vi "Servo(s) (subVI).vi"(0 "PWM channel 2":tag="B/PWM0", 2 "duty cycle [%]":dbl, 3 "error in (no error)":errorcluster) -> (10 "error out":errorcluster)   [LabVIEW 2017]
uses:
  <vilib>/Utility/error.llb/Error Cluster From Error Code.vi
  <vilib>/myRIO/Instrument Drivers/Onboard IO/PWM/PWM.lvlib
panel:
  in  "Servo stop":bool
  in  "freq [Hz]":dbl=50.0
  # "Servo"
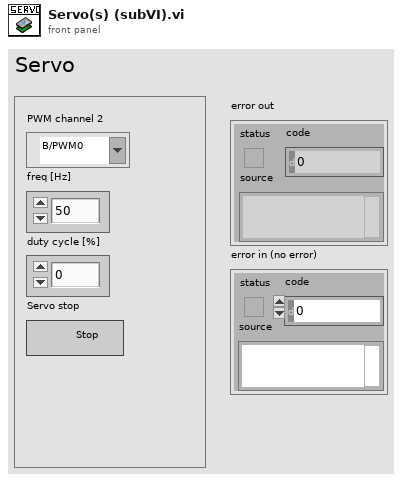
[diagram p1: front panel]
types:
  T1 = typedef "PWM.lvlib/PWM Reference.ctl" = cluster{"myRIO Reference":T2, "PWM Channels Enum":T6, "PWM Configuration":T7}
  T2 = typedef "myRIO Generic Hardware Reference.ctl" = cluster{"myRIO Model":T3, "myRIO Hardware Reference":T4}
  T3 = typedef "Hardware Version Enum.ctl" = enum16{"Unknown", "myRIO-1900", "myRIO-1950", "roboRIO", "NI ELVIS RIO CM"}
  T4 = typedef "myRIO v1.0 Reference.ctl" = cluster{"Generic FPGA Reference":T5, "Allow multiple opens":bool}
  T5 = typedef "Generic FPGA Reference.ctl" = refnum<k20>
  T6 = typedef "PWM Channels Enum.ctl" = enum16{"Not Connected", "C/PWM0", "C/PWM1", "A/PWM0", "A/PWM1", "A/PWM2", "B/PWM0", "B/PWM1", "B/PWM2", "PWM/PWM0", "PWM/PWM1", "PWM/PWM2", "PWM/PWM3", "PWM/PWM4", "PWM/PWM5", "PWM/PWM6", "PWM/PWM7", "PWM/PWM8", "PWM/PWM9"}
  T7 = typedef "PWM.lvlib/PWM Configuration.ctl" = cluster{"Frequency":dbl, "Duty Cycle":dbl}
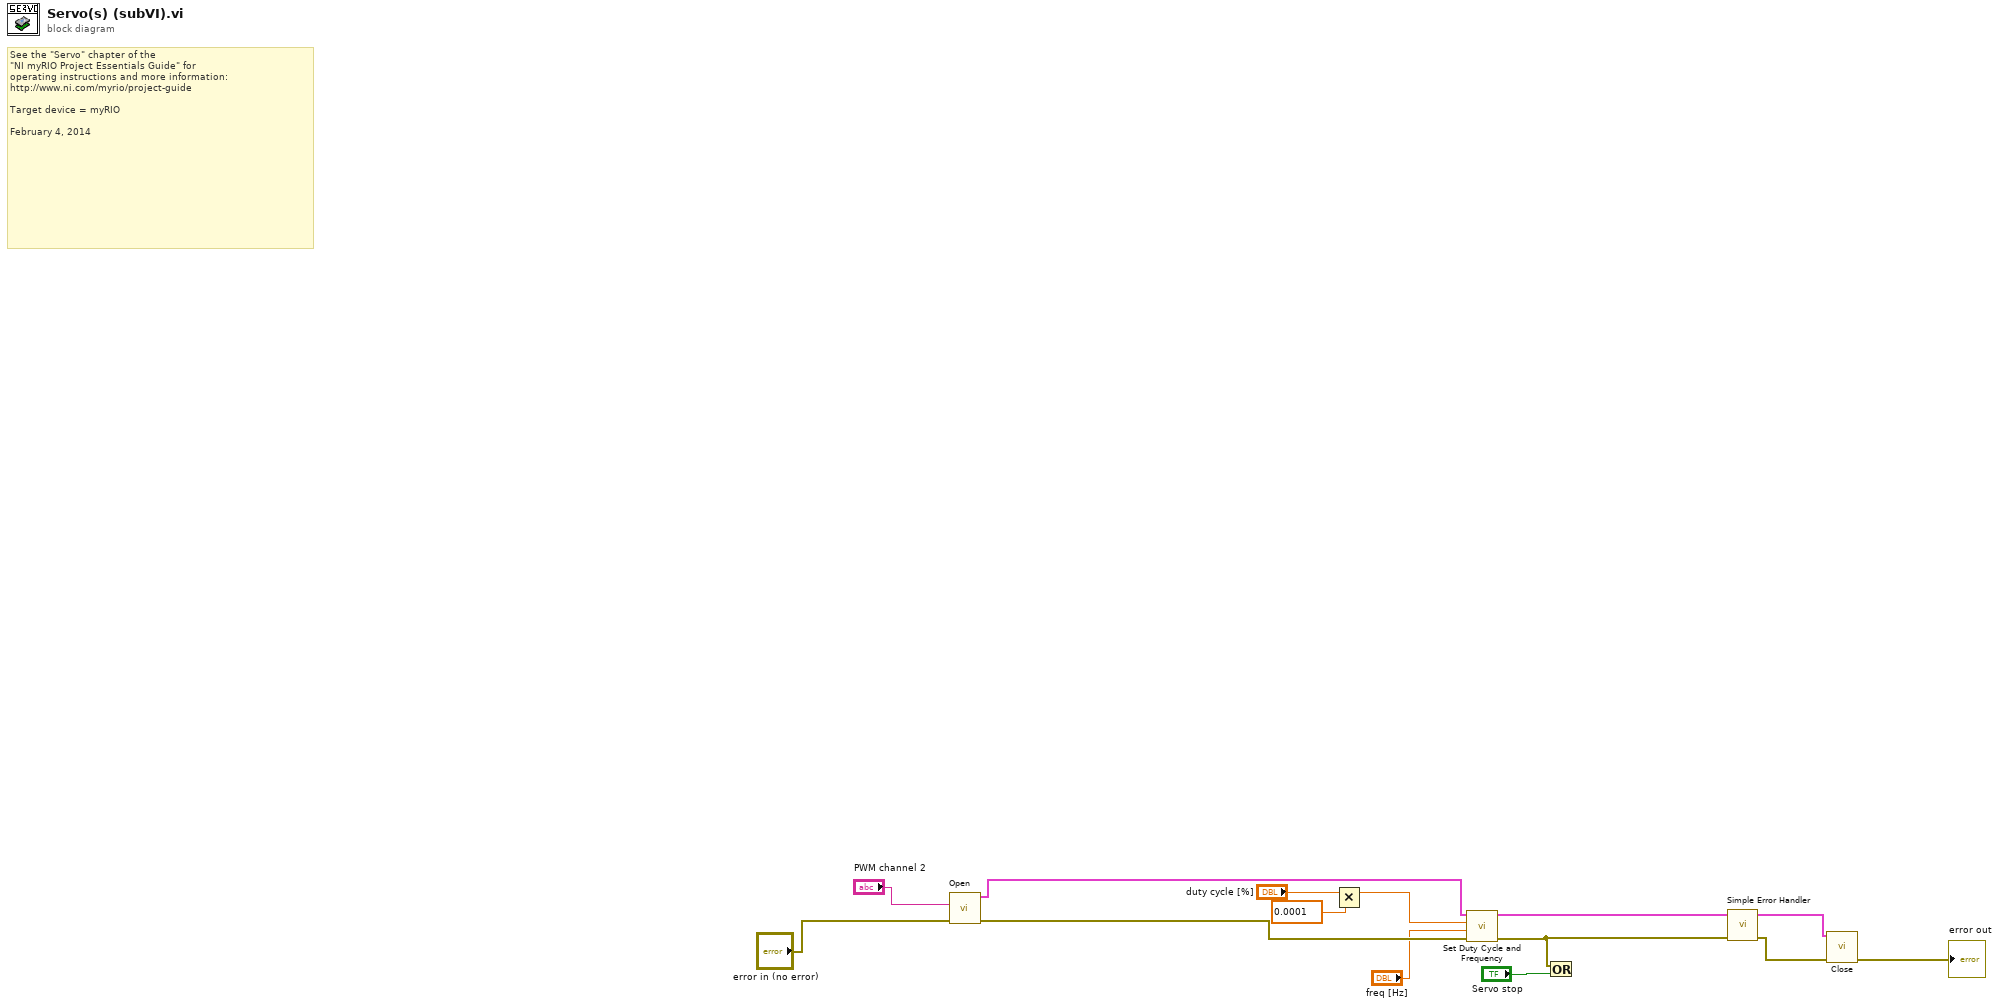
[diagram p0: block diagram]
diagram:
  # "See the \"Servo\" chapter of the\n\"NI myRIO Project Essentials Guide\" for\noperating instructions and more information: \nhttp://www.ni.com/myrio/project-guide\n\nTarget device = myRIO\n\nFebruary 4, 2014"
  n1 = call <vilib>:"Open.vi"("error in (no error)"="error in (no error)", "Channel Name"="PWM channel 2") -> ("error out"=w7:errorcluster, "PWM Ref Out"=w6:T1)  [unwired: 8 in]
  n2 = Multiply(x="duty cycle [%]", y=0.0001) -> (x*y=w2:dbl)
  n3 = call <vilib>:"Set Duty Cycle and Frequency.vi"("error in (no error)"=w7, "Frequency [Hz]"="freq [Hz]", "Duty Cycle"=w2, "PWM Ref In"=w6) -> ("error out"=w10:errorcluster, "PWM Ref Out"=w11:T1)  [unwired: 5 in]
  n4 = Or(x=w10, y="Servo stop") -> ()  [unwired: 1 out]
  n5 = call <vilib>:"Simple Error Handler.vi"("error in (no error)"=w10) -> ("error out"=w13:errorcluster)  [unwired: 4 in, 4 out]
  n6 = call <vilib>:"Close.vi"("error in (no error)"=w13, "PWM Ref In"=w11) -> ("error out"=→"error out":errorcluster)  [unwired: 9 in]
